vi "Test Parallel Logic.vi"() -> ()   [LabVIEW 2021]
uses:
  Source/Support/Nodes/abs_Node/Status.ctl
  Source/Support/Nodes/Composites/abs_Parallel/Support/Status Calculation.ctl
  Source/Support/Nodes/Composites/abs_Parallel/bt_Parallel.lvclass
  Source/Support/Nodes/abs_Node/bt_Node.lvclass
panel:
  in  "stop":bool
  in  "Status Calculation":T1
  out "Status":T2
  in  "Array":T2[](array[typedef])
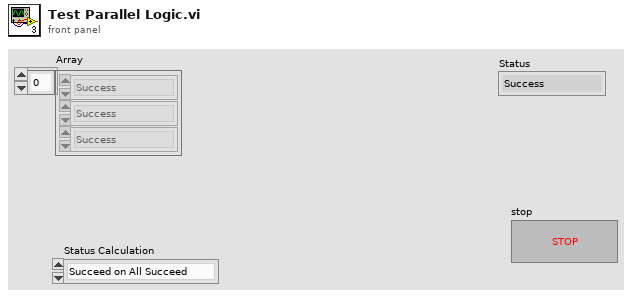
[diagram p1: front panel]
types:
  T1 = typedef "BT.lvlib/bt_Parallel.lvclass/Status Calculation.ctl" = enum16{"Succeed on All Succeed", "Failure on All Failure", "Succeed on Any Succeed", "Failure on Any Failure"}
  T2 = typedef "BT.lvlib/bt_Node.lvclass/Status.ctl" = enum16{"Success", "Failure", "Running"}
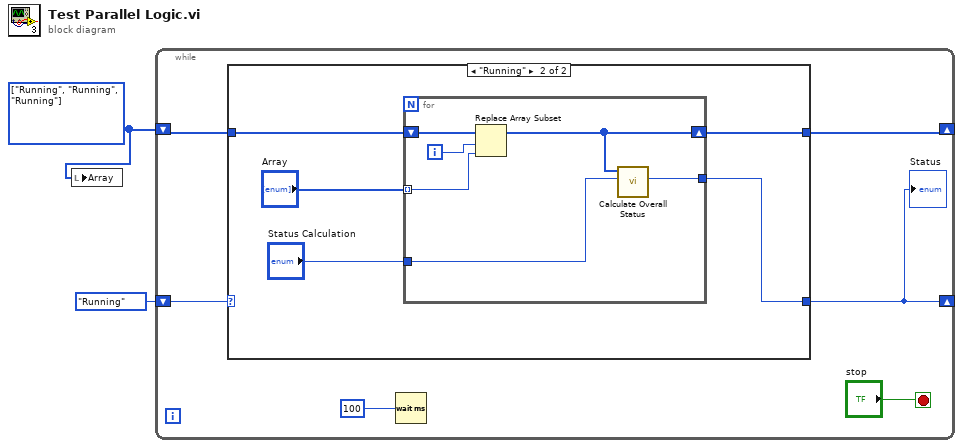
[diagram p0: block diagram]
diagram:
  w2 = T2[] [enum."Running", enum."Running", enum."Running"] items=["Success", "Failure", "Running"] ("Array")
  n1 = local write "Array"(w2) -> ()
  n2 = while {
    shift-right: [w5] -> _
    shift-left: w2 -> [w6]
    shift-right: [w3] -> _
    shift-left: Status."Running" ("Overall Status") -> [w4]
    stop <- "stop" stop-if-true
    n3 = case shown="\"Running\"" w4 {
      selector: w4 -> [w9 _]
      tunnel: w6 -> [w10 w13]
      tunnel: [w10 w12] -> w5
      tunnel: [w9 w11] -> w3
      frame Default {
      }
      frame "Running" {
        n4 = for {
          tunnel: "Array" -> [w20] mode=indexing
          tunnel: "Status Calculation" -> [w21]
          shift-right: [w18] -> w12
          shift-left: w13 -> [w19]
          tunnel: [w17] -> w11
          i -> [w16]
          n5 = Replace Array Subset(array=w19, new element=w20, index=w16) -> (w18:T2[])
          n6 = call "Calculate Overall Status.vi"("Status Calculation"=w21, "Status's"=w18) -> ("Overall Status"=w17:T2)  [unwired: 9 in]
        }
      }
    }
    "Status" <- w3
    n7 = Wait (ms)(milliseconds to wait=u32 100) -> ()  [unwired: 1 out]
  }
